vi "array_speedmode.vi"(2 "# of points":i32, 3 "indep array (x) in":dbl[](array[numeric])) -> (0 "extracted data":dbl[](array[numeric]))   [LabVIEW 2020]
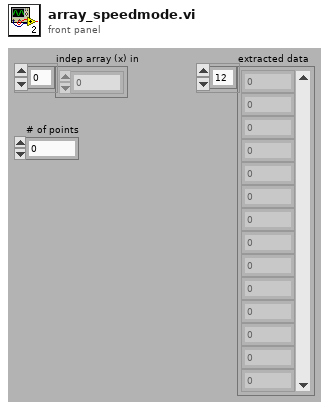
[diagram p1: front panel]
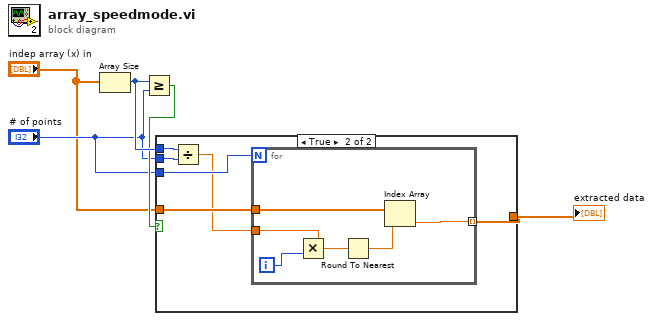
[diagram p0: block diagram]
diagram:
  n1 = Array Size(array="indep array (x) in") -> (size(s)=w4:i32)
  n2 = Greater Or Equal?(x=w4, y="# of points") -> (x >= y?=w3:bool)
  n3 = case shown="True" w3 {
    tunnel: "indep array (x) in" -> [w6 w10]
    tunnel: [w6 w9] -> w5
    tunnel: w4 -> [_ w12]
    tunnel: "# of points" -> [_ w11]
    tunnel: "# of points" -> [_ w8]
    frame False {
    }
    frame True {
      n4 = Divide(x=w12, y=w11) -> (x/y=w7:dbl)
      n5 = for {
        N: w8 -> [_]
        tunnel: w10 -> [w18]
        tunnel: [w17] -> w9 mode=indexing
        tunnel: w7 -> [w16]
        i -> [w15]
        n6 = Multiply(x=w16, y=w15) -> (x*y=w14:dbl)
        n7 = Round To Nearest(number=w14) -> (nearest integer value=w13:dbl)
        n8 = Index Array(array=w18, index=w13) -> (element=w17:dbl)
      }
    }
  }
  "extracted data" <- w5
